vi "Initialize Instrument.vi"(8 "error in (no error)":errorcluster, 10 "Instr Resource Str":string, 11 "NI Sig Gen.lvclass in":refnum<class "NI Sig Gen.lvclass">) -> (0 "error out":errorcluster, 3 "NI Sig Gen.lvclass out":refnum<class "NI Sig Gen.lvclass">)   [LabVIEW 2011, in "NI Sig Gen.lvclass"]
uses:
  NI Sig Gen.lvclass
  NI Sig Gen.lvclass/NI Sig Gen.ctl
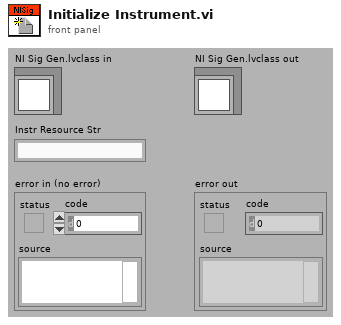
[diagram p1: front panel]
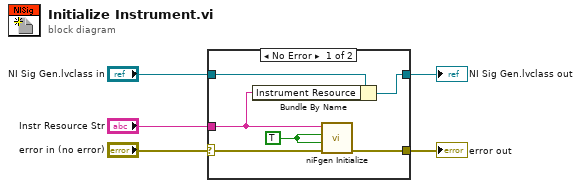
[diagram p0: block diagram]
diagram:
  n1 = case shown="No Error" "error in (no error)" {
    selector: "error in (no error)" -> [w10 w12]
    tunnel: [w7 w13] -> w4
    tunnel: [w9 w12] -> w5
    tunnel: "NI Sig Gen.lvclass in" -> [w8 w13]
    tunnel: "Instr Resource Str" -> [w6 _]
    frame No Error {
      w11 = TRUE ("ID Query? (T: Yes)")
      n2 = Bundle By Name(cluster=w8, "Instrument Resource"=w6) -> (w7:refnum<class "NI Sig Gen.lvclass">)
      n3 = call <instrlib>:"niFgen Initialize.vi"("error in (no error)"=w10, "Reset Device (default: True)"=w11, "Id Query (default: True)"=w11, "Resource Name"=w6) -> ("error out"=w9:errorcluster)  [unwired: 7 out]
    }
    frame Error {
    }
  }
  "error out" <- w5
  "NI Sig Gen.lvclass out" <- w4
